vi "BM_heat_test_subVI.vi"(5 "error in (no error)":errorcluster, 8 "Heat Pulse Delay (ms)":u32=1000, 9 "Trap Heating Time (ms)":i32=700, 10 "BitNum":u32=1, 11 "BoardNum":u32) -> (0 "Heating trap worked!":bool=TRUE, 1 "Final Temp (c)":sgl=44.220646, 2 "Initial Temp (c)":sgl=37.116043, 3 "HEATING!!":bool, 4 "error out":errorcluster)   [LabVIEW 2021]
uses:
  GLOBAL_heating_indicator.vi
panel:
  # "BitNum:\nOSSCAR = 1\nPeTeR = 0"
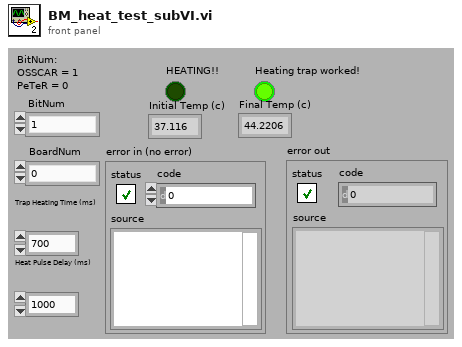
[diagram p1: front panel]
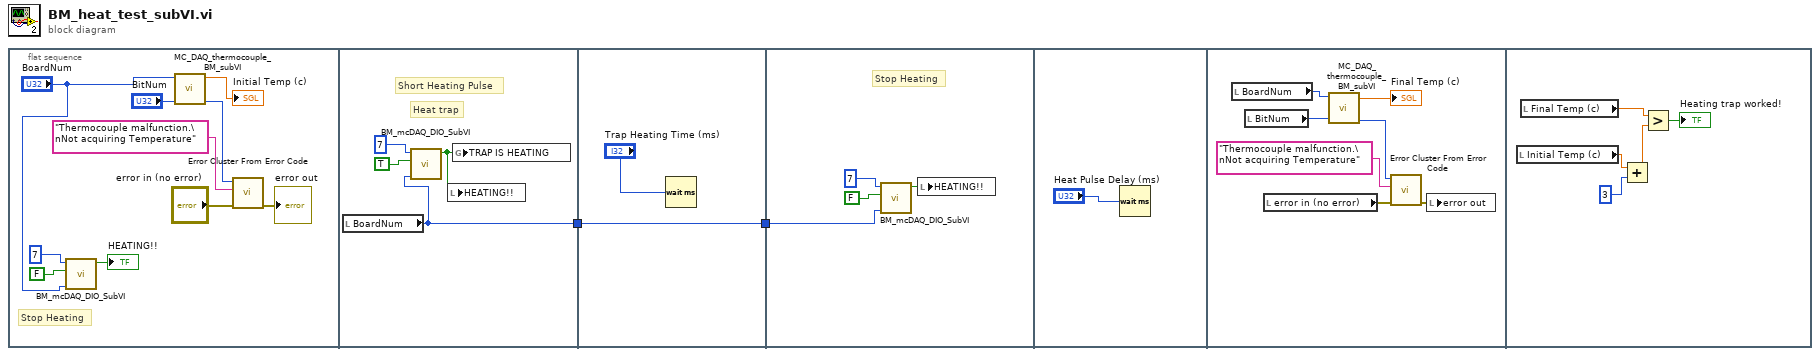
[diagram p0: block diagram]
diagram:
  n1 = flat-sequence {
    tunnel: [w13] -> w1
    tunnel: [w17] -> w2
    tunnel: w1 -> [w17]
    tunnel: w2 -> [w19]
    frame #0 {
      # "Stop Heating"
      n2 = call "BM_mcDAQ_DIO_SubVI.vi"("BoardNum"="BoardNum", "BitValue"=FALSE, "BitNum"=7) -> ("Control out"=→"HEATING!!":bool)  [unwired: 8 in]
      n3 = call "MC_DAQ_thermocouple_BM_subVI.vi"("BitNum"="BitNum", "BoardNum"="BoardNum") -> ("Error code"=w6:i32, "Temp (oC)"=→"Initial Temp (c)":dbl)  [unwired: 8 in]
      n4 = call <vilib>:"Error Cluster From Error Code.vi"("error in (no error)"="error in (no error)", "error message (\"\")"="Thermocouple malfunction.\nNot acquiring Temperature", "error code (0)"=w6) -> ("error out"=→"error out":errorcluster)  [unwired: 1 in, 5 out]
    }
    frame #1 {
      # "Short Heating Pulse"
      # "Heat trap"
      n5 = local read "BoardNum"() -> (w13:u32)
      n6 = call "BM_mcDAQ_DIO_SubVI.vi"("BoardNum"=w13, "BitValue"=TRUE, "BitNum"=7) -> ("Control out"=w14:bool)  [unwired: 8 in]
      n7 = local write "HEATING!!"(w14) -> ()
      n8 = global write "GLOBAL_heating_indicator.vi" "TRAP IS HEATING"(w14) -> ()
    }
    frame #2 {
      n9 = Wait (ms)(milliseconds to wait="Trap Heating Time (ms)") -> ()  [unwired: 1 out]
    }
    frame #3 {
      # "Stop Heating"
      n10 = call "BM_mcDAQ_DIO_SubVI.vi"("BoardNum"=w19, "BitValue"=FALSE, "BitNum"=7) -> ("Control out"=w20:bool)  [unwired: 8 in]
      n11 = local write "HEATING!!"(w20) -> ()
    }
    frame #4 {
      n12 = Wait (ms)(milliseconds to wait="Heat Pulse Delay (ms)") -> ()  [unwired: 1 out]
    }
    frame #5 {
      n13 = local read "BoardNum"() -> (w25:u32)
      n14 = local read "BitNum"() -> (w24:u32)
      n15 = local read "error in (no error)"() -> (w29:errorcluster)
      n16 = call "MC_DAQ_thermocouple_BM_subVI.vi"("BitNum"=w24, "BoardNum"=w25) -> ("Error code"=w26:i32, "Temp (oC)"=→"Final Temp (c)":dbl)  [unwired: 8 in]
      n17 = call <vilib>:"Error Cluster From Error Code.vi"("error in (no error)"=w29, "error message (\"\")"="Thermocouple malfunction.\nNot acquiring Temperature", "error code (0)"=w26) -> ("error out"=w28:errorcluster)  [unwired: 1 in, 5 out]
      n18 = local write "error out"(w28) -> ()
    }
    frame #6 {
      n19 = local read "Initial Temp (c)"() -> (w32:sgl)
      n20 = local read "Final Temp (c)"() -> (w34:sgl)
      n21 = Add(x=w32, y=3) -> (x+y=w31:sgl)
      n22 = Greater?(x=w34, y=w31) -> (0:→"Heating trap worked!":bool)
    }
  }
